vi "Write Camera Status.vi"(8 "error in (no error)":errorcluster, 10 "Camera Status":T1, 11 "Construct String Camera Status in":refnum<class "Construct String Camera Status.lvclass">) -> (0 "error out":errorcluster, 3 "Construct String Camera Status out":refnum<class "Construct String Camera Status.lvclass">)   [LabVIEW 2018, in "Construct String Camera Status.lvclass"]
doc: "Este VI recebe um cluster contendo o status da câmera, escrevendo estas informações na classe."
uses:
  Construct String Camera Status.lvclass
  Construct String Camera Status.lvclass/Construct String Camera Status.ctl
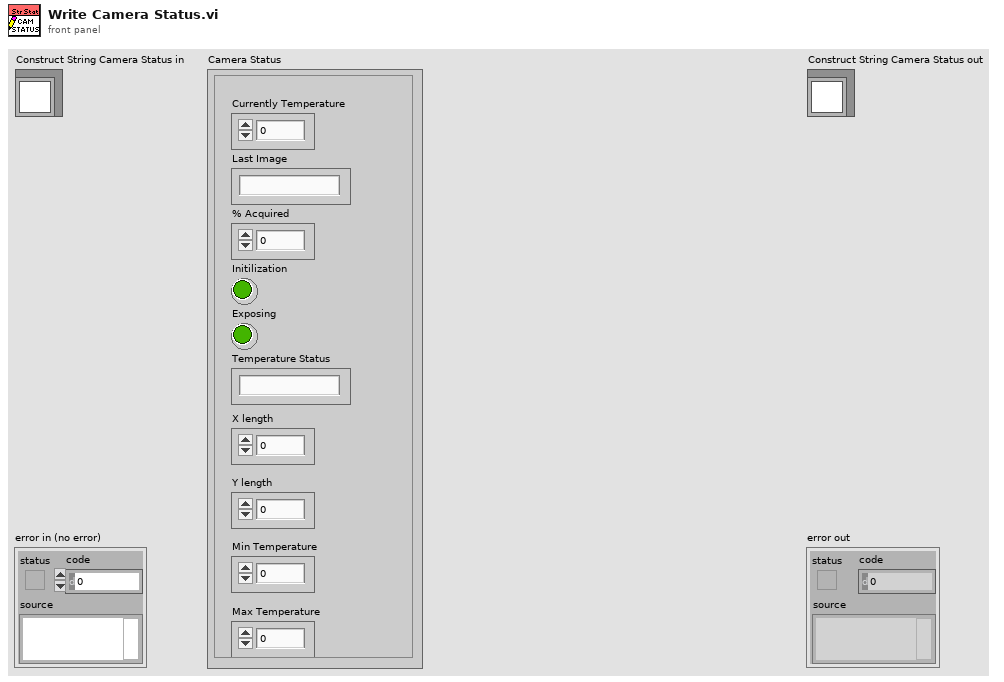
[diagram p1: front panel]
types:
  T1 = cluster{"Currently Temperature":dbl, "Last Image":string, "% Acquired":dbl, "Initilization":bool, "Exposing":bool, "Temperature Status":string, "X length":dbl, "Y length":dbl, "Min Temperature":dbl, "Max Temperature":dbl}
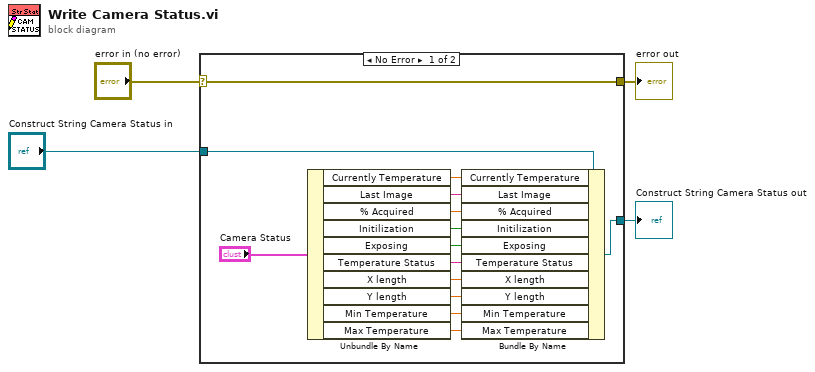
[diagram p0: block diagram]
diagram:
  n1 = case shown="No Error" "error in (no error)" {
    selector: "error in (no error)" -> [w18 w19]
    tunnel: [w18 w19] -> w3
    tunnel: [w17 w20] -> w1
    tunnel: "Construct String Camera Status in" -> [w16 w20]
    frame No Error {
      n2 = Unbundle By Name("Camera Status") -> ("Currently Temperature"=w10:dbl, "Last Image"=w11:string, "% Acquired"=w12:dbl, "Initilization"=w13:bool, "Exposing"=w14:bool, "Temperature Status"=w15:string, "X length"=w5:dbl, "Y length"=w6:dbl, "Min Temperature"=w7:dbl, "Max Temperature"=w8:dbl)
      n3 = Bundle By Name(cluster=w16, "Currently Temperature"=w10, "Last Image"=w11, "% Acquired"=w12, "Initilization"=w13, "Exposing"=w14, "Temperature Status"=w15, "X length"=w5, "Y length"=w6, "Min Temperature"=w7, "Max Temperature"=w8) -> (w17:refnum<class "Construct String Camera Status.lvclass">)
    }
    frame Error {
    }
  }
  "error out" <- w3
  "Construct String Camera Status out" <- w1
